vi "Get Picture.vi"(8 "error in (no error)":errorcluster, 11 "LED Matrix in":refnum<class "LED Matrix.lvclass">) -> (0 "error out":errorcluster, 2 "Picture":picture, 3 "LED Matrix out":refnum<class "LED Matrix.lvclass">)   [LabVIEW 2020, in "LED Matrix.lvclass"]
uses:
  LED Matrix.lvclass
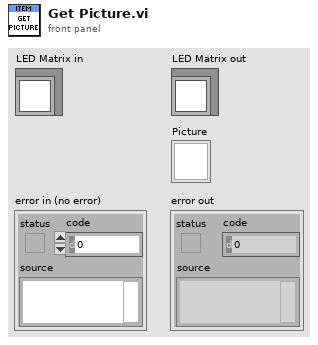
[diagram p1: front panel]
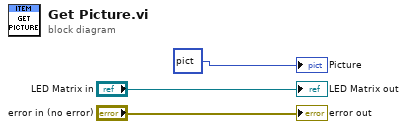
[diagram p0: block diagram]
diagram:
  "error out" <- "error in (no error)"
  "LED Matrix out" <- "LED Matrix in"
  "Picture" <- picture bytes[3230] ("new picture")
